vi "pp_ColorArrayToMixed.vi"(0 "Array In":u32[](array[colorbox])) -> (1 "Value":u32(colorbox), 2 "Mixed?":bool)   [LabVIEW 2017]
doc: "Tells you (with the boolean) if the array contains mixed values, and if they're all the same value, what that value is (with the output color)."
panel:
  # "Tells you (with the boolean) if the array contains mixed values, and\nif they're all the same value, what that value is (with the output color)."
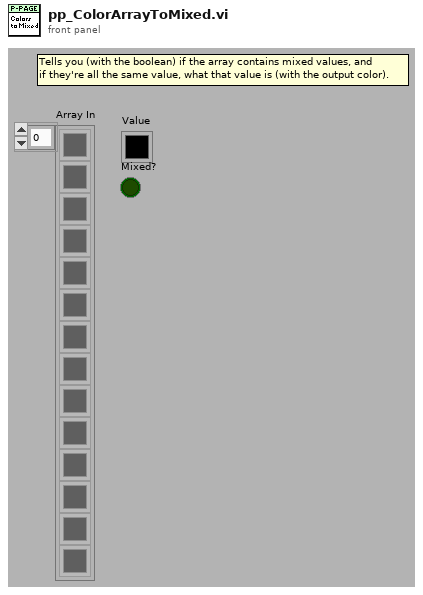
[diagram p1: front panel]
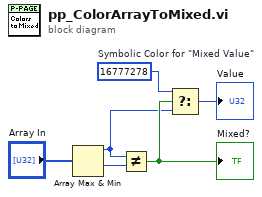
[diagram p0: block diagram]
diagram:
  w2 = u32 16777278  # Symbolic Color for "Mixed Value"
  n1 = Array Max & Min(array="Array In") -> (max value=w3:u32, min value=w5:u32)  [unwired: 2 out]
  n2 = Not Equal?(x=w3, y=w5) -> (x != y?=w4:bool)
  "Mixed?" <- w4
  n3 = Select(t=w2, s=w4, f=w3) -> (s? t:f=→"Value":u32)
